vi "IMAQdx Write Register.vi"(8 "error in":errorcluster, 9 "Value":u32 format="%.0x", 10 "Offset":u32=4042262528 format="%.0x", 11 "Session In":T1) -> (0 "error out":errorcluster, 3 "Session Out":T1)   [LabVIEW 2020, in "NI_Vision_Acquisition_Software.lvlib"]
doc: "Accesses registers on the camera and writes a 32-bit value to the camera. Data is byte-swapped for big endian alignment before transfer."
uses:
  NI_Vision_Acquisition_Software.lvlib
  IMAQdx.ctl
  niimaqdx.dll
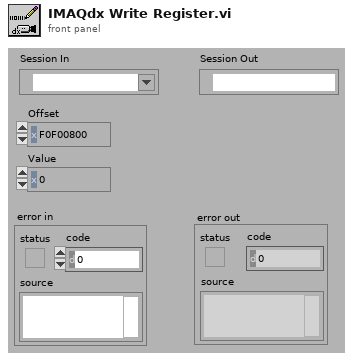
[diagram p1: front panel]
types:
  T1 = typedef "IMAQdx.ctl" = refnum<k21>
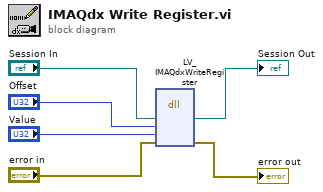
[diagram p0: block diagram]
diagram:
  n1 = dll-call lib="niimaqdx.dll" fn="LV_IMAQdxWriteRegister"("Session In"="Session In", "offset"="Offset", "value"="Value", "error in"="error in") -> ("Session In"=→"Session Out":T1, "error in"=→"error out":errorcluster)  [unwired: 6 in, 2 out]
